vi "Vision Research Phantom Series PhCon PhAddSimulatedCamera.vi"(0 "CamVer (in)":u32=1, 2 "Serial (in)":u32=1, 5 "Error In (no error)":errorcluster) -> (19 "Error Out":errorcluster)   [LabVIEW 2013, in "VRI.lvlib"]
doc: "PhCon.dll\n\nPhAddSimulatedCamera\nHRESULT PhAddSimulatedCamera(UINT CamVer, UINT Serial)\n\nParameters Description\nCamVer (in) Simulated camera version.\nSerial (in) The serial you want for the simulated camera.\nReturn HRESULT (0 = Ok)\nComments Add a new simulated camera to the camera pool.\n PhGetCameraCount will count these cameras too.\n You may later load an stg file for the camera\n having the specified serial and simulate the \n behavior and the calibrations of that camera."
uses:
  VRI.lvlib
  Phantom DLLs/PhCon.dll
panel:
  # "For instructions on the use of this VI, press Ctrl+H to display the help window and move the mouse over the icon, controls, and indicators"
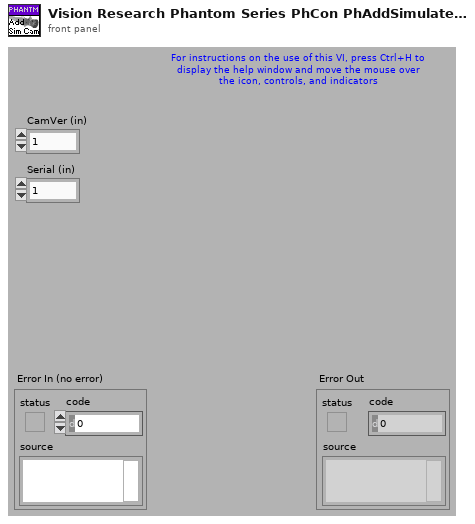
[diagram p1: front panel]
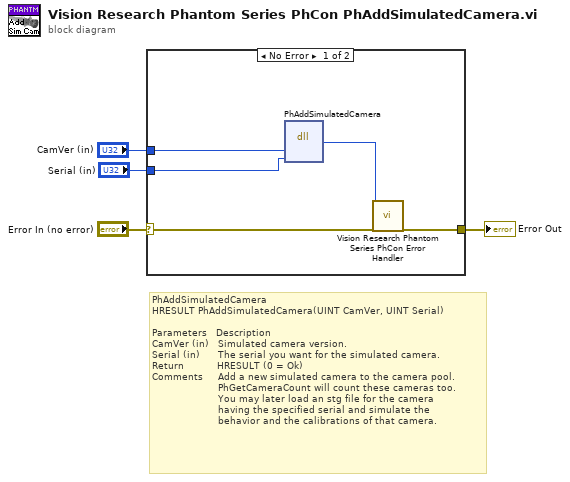
[diagram p0: block diagram]
diagram:
  # "PhAddSimulatedCamera\nHRESULT PhAddSimulatedCamera(UINT CamVer, UINT Serial)\n\nParameters   Description\nCamVer (in)   Simulated camera version.\nSerial (in)      The serial you want for the simulated camera.\nReturn           HRESULT (0 = Ok)\nComments     Add a new simulated camera to the camera pool.\n                      PhGetCameraCount will count these cameras too.\n                      You may later load an stg file for the camera\n                      having the specified serial and simulate the \n                      behavior and the calibrations of that camera."
  n1 = case shown="No Error" "Error In (no error)" {
    selector: "Error In (no error)" -> [w9 w10]
    tunnel: [w8 w10] -> w3
    tunnel: "CamVer (in)" -> [w7 _]
    tunnel: "Serial (in)" -> [w6 _]
    frame No Error {
      n2 = dll-call lib="C:/Projects/SDK/32-bit/Vision Research Phantom Series Labview Driver/Phantom DLLs/PhCon.dll" fn="PhAddSimulatedCamera"("CamVer"=w7, "Serial"=w6) -> ("HRESULT"=w5:i32)  [unwired: 5 in, 2 out]
      n3 = call "Vision Research Phantom Series PhCon Error Handler.vi"("ErrNo"=w5, "Error In (no error)"=w9) -> ("Error Out"=w8:errorcluster)  [unwired: 17 out]
    }
    frame Error {
    }
  }
  "Error Out" <- w3
